vi "Page_Info_Validate_Filename.vi"(8 "error in (no error)":errorcluster, 10 "Filename in":string, 11 "AB_EXE in":refnum<class "AB_EXE.lvclass">) -> (0 "error out":errorcluster, 1 "hasInvalidCharacters":bool, 2 "Filename out":string, 3 "AB_EXE out":refnum<class "AB_EXE.lvclass">, 5 "message":string)   [LabVIEW 2020, in "AB_EXE.lvclass"]
uses:
  <vilib>/AppBuilder/AB_Classes/EXE/AB_EXE.lvclass
  <vilib>/AppBuilder/AB_Classes/Application/AB_Application.lvclass
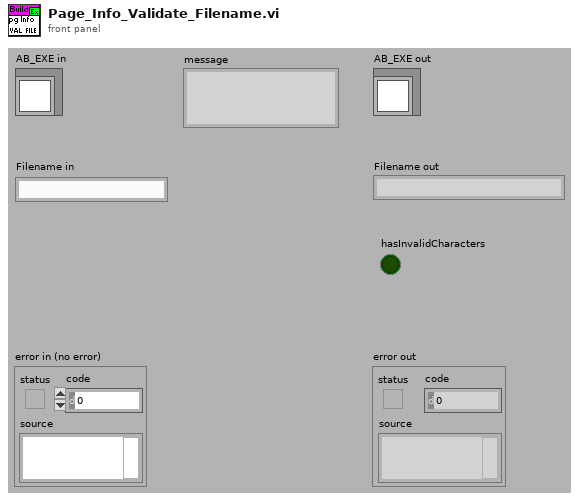
[diagram p1: front panel]
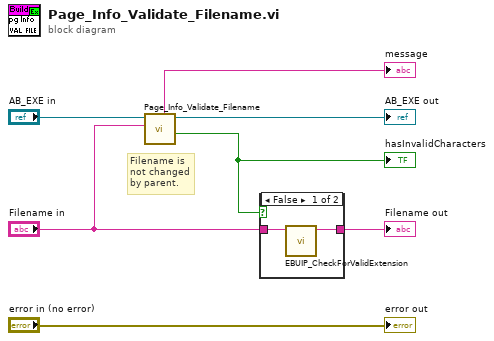
[diagram p0: block diagram]
diagram:
  # "Filename is not changed by parent."
  n1 = call-parent "Page_Info_Validate_Filename.vi"("Filename in"="Filename in", "AB_Targetfile in"="AB_EXE in") -> ("hasInvalidCharacters"=w2:bool, "AB_Targetfile out"=→"AB_EXE out":refnum<class "AB_EXE.lvclass">, "message"=→"message":string)  [unwired: 5 in, 2 out]
  "hasInvalidCharacters" <- w2
  n2 = case shown="False" w2 {
    tunnel: [w8 w10] -> w3
    tunnel: "Filename in" -> [w9 w10]
    frame False {
      n3 = call <resource>:"EBUIP_CheckForValidExtension.vi"("Filename in"=w9) -> ("Filename out"=w8:string)  [unwired: 9 in, 1 out]
    }
    frame True {
    }
  }
  "Filename out" <- w3
  "error out" <- "error in (no error)"
